vi "WM Geometric Settings.vi"(1 "Geometric Settings":T1={"Stroke Calibration"=7.8564, "Water Depth"=2.44, "Paddle Height"=3.3147} {"Paddle Height" min=0.01 format="%.4f"; "Water Depth" min=0.01 format="%.2f"; "Stroke Calibration" format="%.4f"}) -> (0 "Geometric Settings Output":T1={"Stroke Calibration"=7.8564, "Water Depth"=2.44, "Paddle Height"=3.3147} {"Paddle Height" min=0.01 format="%.4f"; "Water Depth" min=0.01 format="%.2f"; "Stroke Calibration" format="%.4f"})   [LabVIEW 2012]
panel:
  in  "OK":bool
  # "m"
  # "m"
  # "V/m"
  # "m"
  # "m"
  # "V/m"
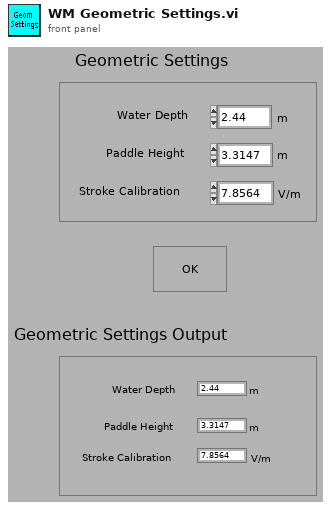
[diagram p1: front panel]
types:
  T1 = cluster{"Stroke Calibration":dbl, "Water Depth":dbl, "Paddle Height":dbl}
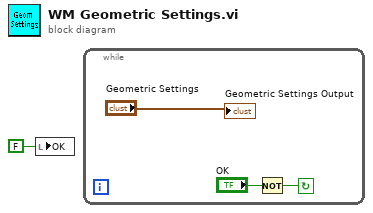
[diagram p0: block diagram]
diagram:
  n1 = local write "OK"(FALSE ("OK")) -> ()
  n2 = while {
    stop <- w2 continue-if-true
    n3 = Not(x="OK") -> (.not. x?=w2:bool)
    "Geometric Settings Output" <- "Geometric Settings"
  }
